vi "VTI test controller.vi"() -> ()   [LabVIEW 2021, in "Temperature controller.lvlib"]
uses:
  Temperature controller.lvlib
  Messenger service/MessengerLib.lvlib
  ctl/MSG for VTI.ctl
  ctl/TC sensors.ctl
  ctl/Set temperature.ctl
  ctl/TC commands.ctl
  ctl/Set point.ctl
panel:
  out "Last message log":string
  out "VTI update":bool
  in  "Stop Button":bool
  in  "Initialize btn":bool
  in  "Set VTI btn":bool
  in  "Set temperature":T1={"VTI space [K]"=70.0, "Sample [K]"=75.0, "Heater3 [K]"=1.8, "Heater4 [K]"=1.8, "Out 1 [%]"=0.0, "Out 2 [%]"=0.0, "Range out 1"=1} {"Range out 1" items=["Off", "Range 1 (On)", "Range 2", "Range 3", "Range 4", "Range 5"]; "Heater4 [K]" min=1.8 max=300.0; "Heater3 [K]" min=1.8 max=300.0; "Sample [K]" min=1.8 max=300.0}
  out "TC sensors [K]":T2={"VTI space"=70.34, "Sample"=75.12, "He pot"=3.82, "Trap"=33.47, "Ambient"=298.41, "SetP_VTI"=70.0, "SetP_Smp"=75.0, "SetP_Pot"=1.8, "SetP_Trap"=1.8, "Range out 1"=1, "Out 1 [%]"=0.0, "Out 2 [%]"=0.0} {"Range out 1" items=["Off", "Range 1 (On)", "Range 2", "Range 3", "Range 4", "Range 5"]}
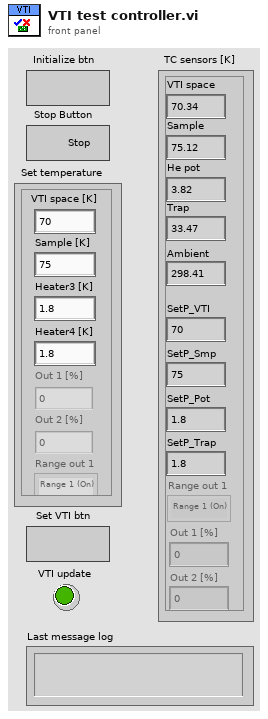
[diagram p1: front panel]
types:
  T1 = typedef "Temperature controller.lvlib/Set temperature.ctl" = cluster{"VTI space [K]":dbl, "Sample [K]":dbl, "Heater3 [K]":dbl, "Heater4 [K]":dbl, "Out 1 [%]":dbl, "Out 2 [%]":dbl, "Range out 1":u16}
  T2 = typedef "Temperature controller.lvlib/TC sensors.ctl" = cluster{"VTI space":dbl, "Sample":dbl, "He pot":dbl, "Trap":dbl, "Ambient":dbl, "SetP_VTI":dbl, "SetP_Smp":dbl, "SetP_Pot":dbl, "SetP_Trap":dbl, "Range out 1":u16, "Out 1 [%]":dbl, "Out 2 [%]":dbl}
  T3 = typedef "MessengerLib.lvlib/Messenger referencies.ctl" = cluster{"TOP":refnum<queue>, "Instr_M":refnum<queue>, "Field_C":refnum<queue>, "Tmp_M":refnum<queue>, "Tmp_C":refnum<queue>, "Table_C":refnum<queue>, "MW_C":refnum<queue>, "Data_Aq":refnum<queue>, "Mod_M":refnum<queue>, "Field_M":refnum<queue>, "Pwr_M":refnum<queue>, "Angle_C":refnum<queue>, "Sample_C":refnum<queue>, "Reserved":refnum<queue>}
  T4 = typedef "Temperature controller.lvlib/MSG for VTI.ctl" = cluster{"Command":T5, "Data":variant}
  T5 = typedef "Temperature controller.lvlib/TC commands.ctl" = enum16{"Initialize", "Update", "Stop tmp change", "Set temperature", "Set point", "Disconnect", "End", "Ignore"}
  T6 = typedef "MessengerLib.lvlib/MSG to TOP.ctl" = cluster{"Module":T7, "Response":string, "Data":variant, "Time":timestamp}
  T7 = typedef "Module name.ctl" = enum16{"Emty", "Magnet", "VTI", "Excitation", "Servo", "Acquisition", "Rotator", "Digitizer", "SMU2450", "Carousel", "Multimeter", "Tmp monitor", "Power monitor"}
  T8 = typedef "Temperature controller.lvlib/Set point.ctl" = cluster{"Heater":string, "Tmp [K]":dbl}
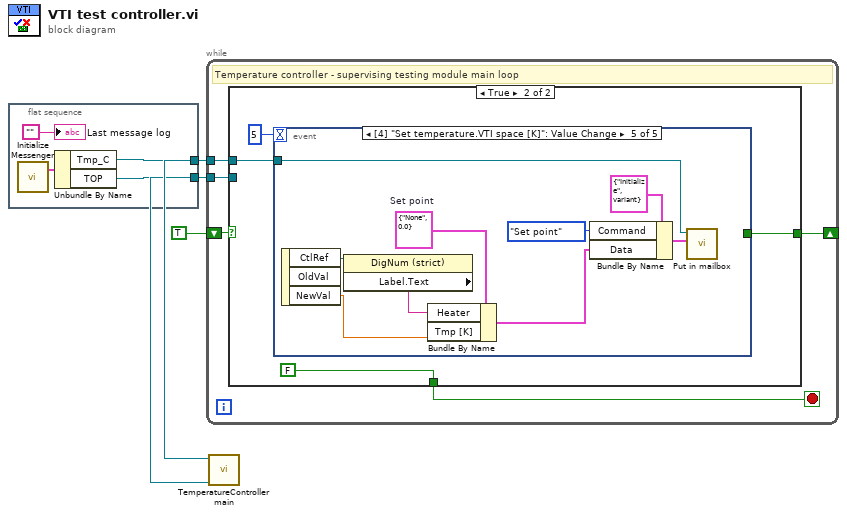
[diagram p0: block diagram]
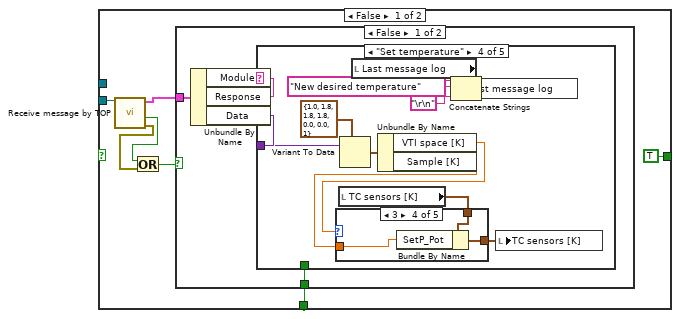
[diagram p2: hidden frame]
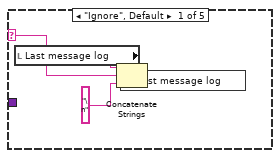
[diagram p3: hidden frame]
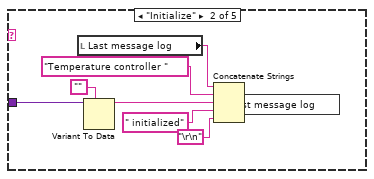
[diagram p4: hidden frame]
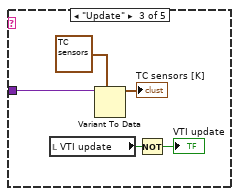
[diagram p5: hidden frame]
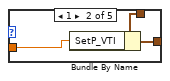
[diagram p7: hidden frame]
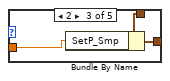
[diagram p8: hidden frame]
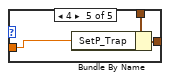
[diagram p9: hidden frame]
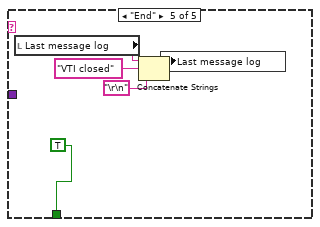
[diagram p10: hidden frame]
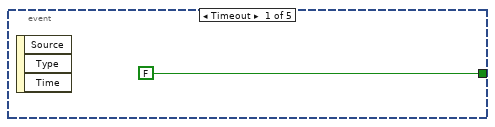
[diagram p12: hidden frame]
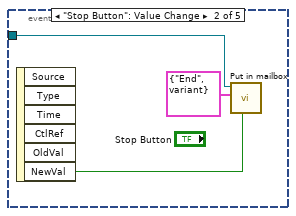
[diagram p13: hidden frame]
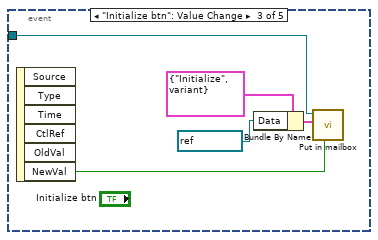
[diagram p14: hidden frame]
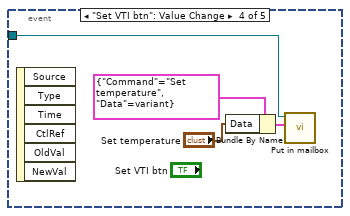
[diagram p15: hidden frame]
diagram:
  n1 = flat-sequence {
    tunnel: [w6] -> w2
    tunnel: [w5] -> w1
    frame #0 {
      n2 = call "Initialize Messenger.vi"() -> ("Referencies out"=w7:T3)  [unwired: 2 in, 1 out]
      n3 = Unbundle By Name(w7) -> ("Tmp_C"=w6:refnum<queue>, "TOP"=w5:refnum<queue>)
      "Last message log" <- ""
    }
  }
  n4 = while {
    shift-right: [w10] -> _
    shift-left: TRUE -> [w11]
    tunnel: w2 -> [w9]
    tunnel: w1 -> [w8]
    stop <- w12 stop-if-true
    # "Temperature controller - supervising testing module main loop"
    n5 = case shown="True" w11 {
      tunnel: [w17 FALSE] -> w12
      tunnel: [TRUE w72] -> w10
      tunnel: w9 -> [_ w71]
      tunnel: w8 -> [w18 _]
      frame False {
        n6 = call "Receive message by TOP.vi"("Mailbox in"=w18) -> ("error out"=w13:errorcluster, "timed out?"=w14:bool, "MSG packet"=w19:T6)  [unwired: 7 in, 1 out]
        n7 = Or(x=w14, y=w13) -> (x .or. y?=w15:bool)
        n8 = case shown="False" w15 {
          tunnel: w19 -> [w23 _]
          tunnel: [w20 _] -> w17
          frame False {
            n9 = Unbundle By Name(w23) -> ("Response"=w22:string, "Data"=w21:variant)  [unwired: 1 out]
            n10 = case shown="\"Set temperature\"" w22 {
              selector: w22 -> [w25 _ _ _ _]
              tunnel: w21 -> [_ w35 w37 w51 _]
              tunnel: [_ _ _ _ TRUE] -> w20
              frame "Ignore", Default {
                n11 = local read "Last message log"() -> (w27:string)
                n12 = Concatenate Strings(w27, w25, "\n" ("string")) -> (w24:string)
                n13 = local write "Last message log"(w24) -> ()
              }
              frame "Initialize" {
                n14 = local read "Last message log"() -> (w30:string)
                n15 = Variant To Data(type="", Variant=w35) -> (data=w33:string)  [unwired: 1 in, 1 out]
                n16 = Concatenate Strings(w30, "Temperature controller " ("string"), w33, " initialized" ("string"), "\r\n") -> (w28:string)
                n17 = local write "Last message log"(w28) -> ()
              }
              frame "Update" {
                n18 = local read "VTI update"() -> (w38:bool)
                n19 = Variant To Data(type=T2 {"VTI space"=0.0, "Sample"=0.0, "He pot"=0.0, "Trap"=0.0, "Ambient"=0.0, "SetP_VTI"=0.0, "SetP_Smp"=0.0, "SetP_Pot"=0.0, "SetP_Trap"=0.0, "Range out 1"=1, "Out 1 [%]"=0.0, "Out 2 [%]"=0.0} ("TC sensors [K]"), Variant=w37) -> (data=→"TC sensors [K]":T2)  [unwired: 1 in, 1 out]
                n20 = Not(x=w38) -> (.not. x?=→"VTI update":bool)
              }
              frame "Set temperature" {
                n21 = local read "TC sensors [K]"() -> (w50:T2)
                n22 = Variant To Data(type=T1 {"VTI space [K]"=1.0, "Sample [K]"=1.8, "Heater3 [K]"=1.8, "Heater4 [K]"=1.8, "Out 1 [%]"=0.0, "Out 2 [%]"=0.0, "Range out 1"=1} ("Set temperature"), Variant=w51) -> (data=w47:T1)  [unwired: 1 in, 1 out]
                n23 = local read "Last message log"() -> (w44:string)
                n24 = Unbundle By Name(w47) -> ("VTI space [K]"=w46:dbl, "Sample [K]"=w45:dbl)
                n25 = case shown="3" w46 {
                  tunnel: w50 -> [w52 w55 w58 w61 w64]
                  tunnel: [w52 w54 w57 w60 w63] -> w48
                  tunnel: w45 -> [_ w53 w56 w59 w62]
                  frame 0, Default {
                  }
                  frame 1 {
                    n26 = Bundle By Name(cluster=w55, "SetP_VTI"=w53) -> (w54:T2)
                  }
                  frame 2 {
                    n27 = Bundle By Name(cluster=w58, "SetP_Smp"=w56) -> (w57:T2)
                  }
                  frame 3 {
                    n28 = Bundle By Name(cluster=w61, "SetP_Pot"=w59) -> (w60:T2)
                  }
                  frame 4 {
                    n29 = Bundle By Name(cluster=w64, "SetP_Trap"=w62) -> (w63:T2)
                  }
                }
                n30 = Concatenate Strings(w44, "New desired temperature" ("string"), "\r\n") -> (w43:string)
                n31 = local write "Last message log"(w43) -> ()
                n32 = local write "TC sensors [K]"(w48) -> ()
              }
              frame "End" {
                n33 = local read "Last message log"() -> (w68:string)
                n34 = Concatenate Strings(w68, "VTI closed" ("string"), "\r\n") -> (w65:string)
                n35 = local write "Last message log"(w65) -> ()
              }
            }
          }
          frame True {
          }
        }
      }
      frame True {
        n36 = event shown="[4] \"Set temperature.VTI space [K]\": Value Change" {
          selector: _ -> [_ _ _ _ _]
          dyn-events: _ -> [_ _ _ _ _]
          timeout: 5 -> [_ _ _ _ _]
          tunnel: [FALSE _ _ _ _] -> w72
          tunnel: w71 -> [_ w77 w82 w86 w87]
          event Timeout {
            n37 = event-data() -> ()  [unwired: 1 in, 3 out]
          }
          event "Stop Button": Value Change {
            n38 = event-data() -> ("NewVal"=w75:bool)  [unwired: 1 in, 5 out]
            n39 = call "Put in mailbox.vi"("Priority? (F)"=w75, "Message"=T4 {"Command"=enum."End", "Data"=variant} ("MSG for VTI"), "Queue in"=w77) -> ()  [unwired: 6 in, 3 out]
          }
          event "Initialize btn": Value Change {
            n40 = event-data() -> ("NewVal"=w78:bool)  [unwired: 1 in, 5 out]
            n41 = Bundle By Name(cluster=T4 {"Command"=enum."Initialize", "Data"=variant} ("MSG for VTI"), "Data"=refnum<visa-resource-name> "COM4" ("VISA resource name")) -> (w80:T4)
            n42 = call "Put in mailbox.vi"("Priority? (F)"=w78, "Message"=w80, "Queue in"=w82) -> ()  [unwired: 6 in, 3 out]
          }
          event "Set VTI btn": Value Change {
            n43 = event-data() -> ()  [unwired: 1 in, 6 out]
            n44 = Bundle By Name(cluster=T4 {"Command"=enum."Set temperature", "Data"=variant} ("MSG for VTI"), "Data"="Set temperature") -> (w84:T4)
            n45 = call "Put in mailbox.vi"("Message"=w84, "Queue in"=w86) -> ()  [unwired: 7 in, 3 out]
          }
          event Value Change {
            w91 = T8 {"Heater"="None", "Tmp [K]"=0.0}  # Set point
            n46 = event-data() -> ("CtlRef"=w89:refnum<vi>, "NewVal"=w88:dbl)  [unwired: 1 in, 1 out]
            n47 = property class="DigNum (strict)"(reference=w89) -> ("Label.Text"=w93:string)  [unwired: 1 in, 2 out]
            n48 = Bundle By Name(cluster=w91, "Heater"=w93, "Tmp [K]"=w88) -> (w90:T8)
            n49 = Bundle By Name(cluster=T4 {"Command"=enum."Initialize", "Data"=variant}, "Command"=TC_commands."Set point", "Data"=w90) -> (w94:T4)
            n50 = call "Put in mailbox.vi"("Message"=w94, "Queue in"=w87) -> ()  [unwired: 7 in, 3 out]
          }
        }
      }
    }
  }
  n51 = call "TemperatureController main.vi"("Supervising module"=w1, "Controller module"=w2) -> ()  [unwired: 10 in]
